vi "Autonomous Independent.vi"   [LabVIEW 2015]
doc: "This VI is called when autonomous begins, and will automatically be terminated when autonomous ends. You can carry out timed or sensor driven robot movement independently without needing to return to the caller."
uses:
  <vilib>/Rock Robotics/WPI/Solenoid/WPI_SolenoidValue.ctl
  <vilib>/Rock Robotics/WPI/Utilities/WPI_GetSetVariantRefNum.vi
  <vilib>/Rock Robotics/Network Tables/NT Read String.vi
  <vilib>/Rock Robotics/Network Tables/NT Read Number.vi
  <vilib>/Rock Robotics/WPI/Solenoid/WPI_SolenoidSetEnum.vi
  <vilib>/Rock Robotics/Network Tables/NT Write Numeric Array.vi
panel:
  # "Be sure to right-click and choose Data Operations>>Make Current Value default if you want to save the array values with the VI"
types:
  T1 = typedef "WPI_JoystickDevRef.ctl" = cluster{"Device":T2}
  T2 = typedef "WPI_JoystickDeviceEnum.ctl" = enum16{"USB 0", "USB 1", "USB 2", "USB 3", "USB 4", "USB 5"}
  T3 = typedef "WPI_ServoDeviceRef.ctl" = cluster{"DeviceStatus":errorcluster, "PWM Channel":T4, "DeadBand":T5}
  T4 = typedef "FPGA_DIOPWMChannel.ctl" = enum8{"PWM 0", "PWM 1", "PWM 2", "PWM 3", "PWM 4", "PWM 5", "PWM 6", "PWM 7", "PWM 8", "PWM 9", "PWM MXP 0", "PWM MXP 1", "PWM MXP 2", "PWM MXP 3", "PWM MXP 4", "PWM MXP 5", "PWM MXP 6", "PWM MXP 7", "PWM MXP 8", "PWM MXP 9", "Invalid"}
  T5 = typedef "WPI_PWMDeadband.ctl" = cluster{"Name":string, "maxPositivePwm":i32, "minPositivePwm":i32, "centerPwm":i32, "maxNegativePwm":i32, "minNegativePwm":i32, "angularRange":u16}
  T6 = typedef "WPI_SolenoidValue.ctl" = enum16{"Off", "On", "Forward", "Reverse"}
  T7 = typedef "WPI_SwitchDevRef.ctl" = cluster{"DevStatus":errorcluster, "DIO Channel":T8, "CntIndex":T9, "Normally Closed":bool}
  T8 = typedef "FPGA_DIOChannel.ctl" = enum8{"DIO 0", "DIO 1", "DIO 2", "DIO 3", "DIO 4", "DIO 5", "DIO 6", "DIO 7", "DIO 8", "DIO 9", "DIO MXP 0", "DIO MXP 1", "DIO MXP 2", "DIO MXP 3", "DIO MXP 4", "DIO MXP 5", "DIO MXP 6", "DIO MXP 7", "DIO MXP 8", "DIO MXP 9", "DIO MXP 10", "DIO MXP 11", "DIO MXP 12", "DIO MXP 13", "DIO MXP 14", "DIO MXP 15", "Invalid"}
  T9 = typedef "FPGA_CounterCtrSystemIndex.ctl" = enum8{"Ctr 0", "Ctr 1", "Ctr 2", "Ctr 3", "Ctr 4", "Ctr 5", "Ctr 6", "Ctr 7", "Invalid"}
  T10 = typedef "WPI_SolenoidDevRef.ctl" = cluster{"DevStatus":errorcluster, "Pneumatics Control Module":u8, "Forward Solenoid Channel":T11, "Reverse Solenoid Channel":T11}
  T11 = typedef "WPI_SolenoidChannel.ctl" = enum8{"Solenoid 0", "Solenoid 1", "Solenoid 2", "Solenoid 3", "Solenoid 4", "Solenoid 5", "Solenoid 6", "Solenoid 7", "Invalid"}
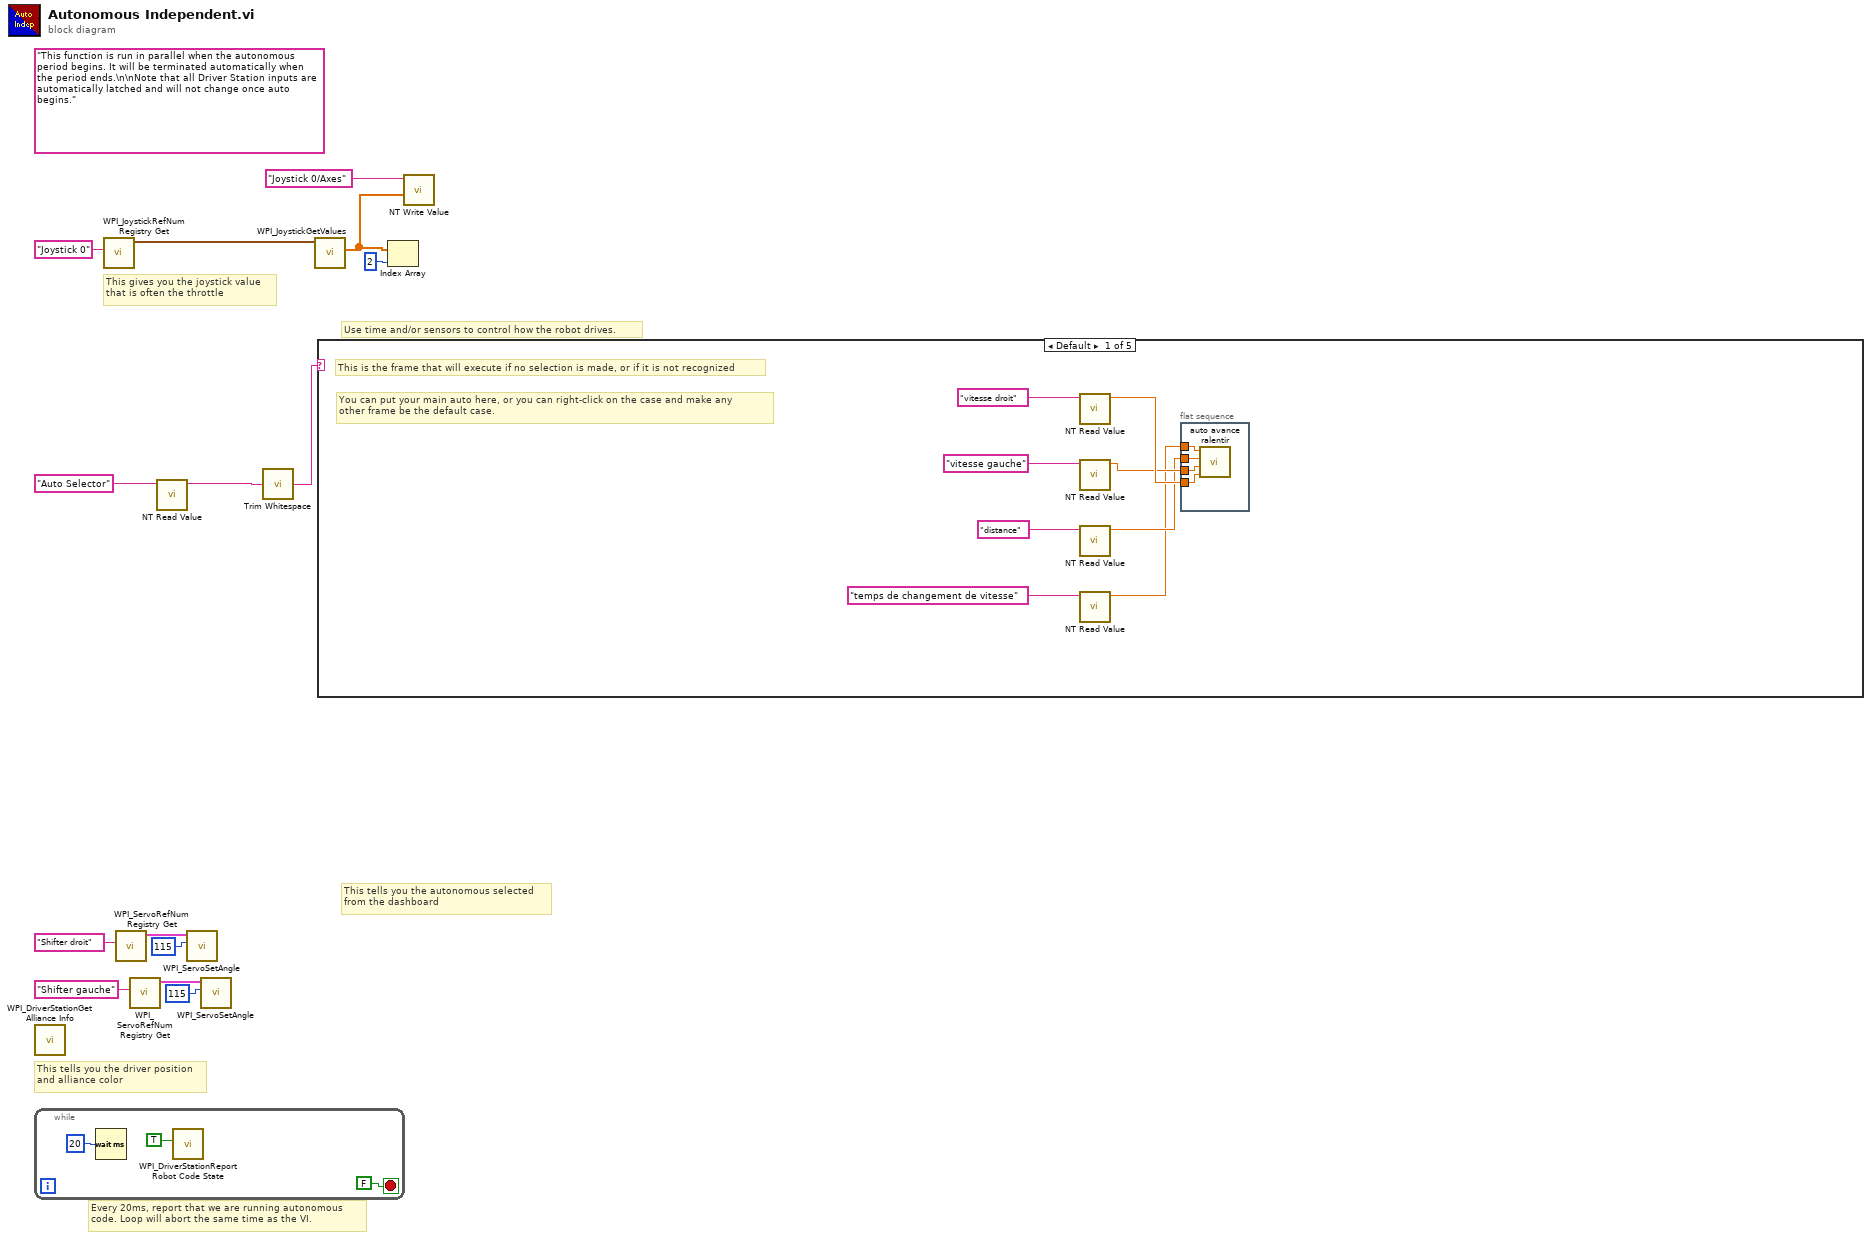
[diagram p0: block diagram]
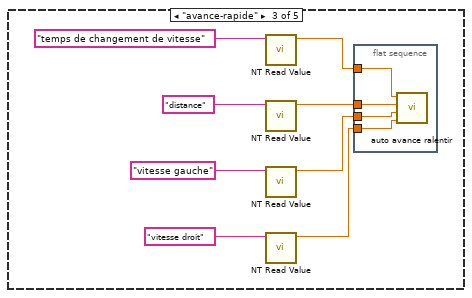
[diagram p3: hidden frame]
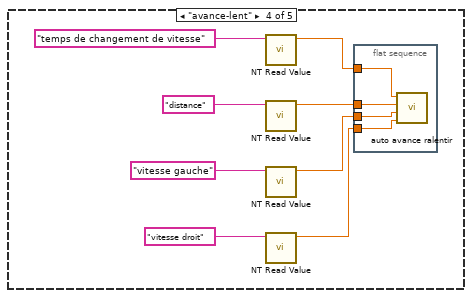
[diagram p4: hidden frame]
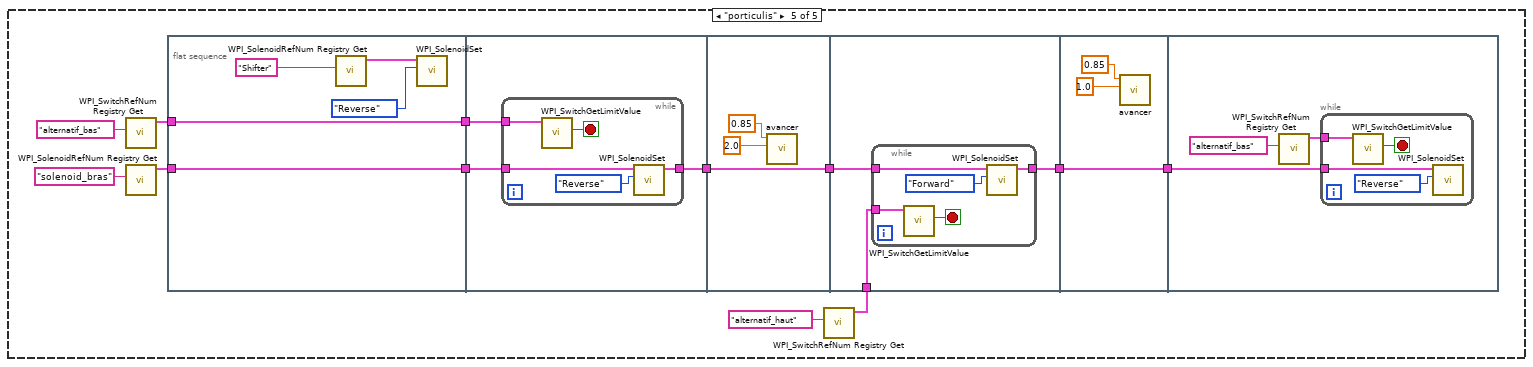
[diagram p5: hidden frame]
diagram:
  (unwired) "This function is run in parallel when the autonomous period begins. It will be terminated automatically when the period ends.\n\nNote that all Driver Station inputs are automatically latched and will not change once auto begins."
  # "This tells you the autonomous selected\nfrom the dashboard"
  # "Every 20ms, report that we are running autonomous\ncode. Loop will abort the same time as the VI."
  # "This gives you the joystick value\nthat is often the throttle"
  # "Use time and/or sensors to control how the robot drives."
  # "This tells you the driver position\nand alliance color"
  n1 = call <vilib>:"WPI_DriverStationGet Alliance Info.vi"() -> ()  [unwired: 12 out]
  n2 = while {
    stop <- FALSE stop-if-true
    n3 = Wait (ms)(milliseconds to wait=u32 20) -> ()  [unwired: 1 out]
    n4 = call <vilib>:"WPI_DriverStationReport Robot Code State.vi"("Autonomous"=TRUE) -> ()  [unwired: 10 in, 1 out]
  }
  n5 = call <vilib>:"WPI_JoystickRefNum Registry Get.vi"("refnum name"="Joystick 0") -> ("JoystickDevRef"=w13:T1)  [unwired: 1 in, 9 out]
  n6 = call <vilib>:"WPI_ServoRefNum Registry Get.vi"("refnum name"="Shifter droit") -> ("ServoDeviceRef"=w5:T3)  [unwired: 9 in, 1 out]
  n7 = call <vilib>:"WPI_ServoRefNum Registry Get.vi"("refnum name"="Shifter gauche") -> ("ServoDeviceRef"=w3:T3)  [unwired: 9 in, 1 out]
  n8 = call-poly <vilib>:"NT Read Value.vi"("Name"="Auto Selector") -> ("String"=w1:string)  [unwired: 9 in, 1 out]
  n9 = call <vilib>:"WPI_ServoSetAngle.vi"("Angle"=115, "ServoDeviceRef"=w5) -> ()  [unwired: 8 in, 2 out]
  n10 = call <vilib>:"WPI_ServoSetAngle.vi"("Angle"=115, "ServoDeviceRef"=w3) -> ()  [unwired: 8 in, 2 out]
  n11 = call <vilib>:"Trim Whitespace.vi"("string"=w1) -> ("trimmed string"=w2:string)  [unwired: 1 in]
  n12 = call <vilib>:"WPI_JoystickGetValues.vi"("JoystickDevRef"=w13) -> ("Axes"=w10:dbl[])  [unwired: 6 in, 4 out]
  n13 = case shown="Default" w2 {
    frame Default {
      # "You can put your main auto here, or you can right-click on the case and make any\nother frame be the default case."
      # "This is the frame that will execute if no selection is made, or if it is not recognized"
      n14 = call-poly <vilib>:"NT Read Value.vi"("Name"="vitesse droit") -> ("Numeric"=w21:dbl)  [unwired: 9 in, 1 out]
      n15 = call-poly <vilib>:"NT Read Value.vi"("Name"="vitesse gauche") -> ("Numeric"=w20:dbl)  [unwired: 9 in, 1 out]
      n16 = call-poly <vilib>:"NT Read Value.vi"("Name"="distance") -> ("Numeric"=w19:dbl)  [unwired: 9 in, 1 out]
      n17 = call-poly <vilib>:"NT Read Value.vi"("Name"="temps de changement de vitesse") -> ("Numeric"=w18:dbl)  [unwired: 9 in, 1 out]
      n18 = flat-sequence {
        tunnel: w18 -> [w29]
        tunnel: w20 -> [w27]
        tunnel: w21 -> [w26]
        tunnel: w19 -> [w28]
        frame #0 {
          n19 = call "auto avance ralentir.vi"("vitesse droit"=w26, "vitesse gauche"=w27, "temps"=w28, "temps de changement de direction"=w29) -> ()  [unwired: 8 in]
        }
      }
    }
    frame "rien" {
    }
    frame "avance-rapide" {
      n20 = call-poly <vilib>:"NT Read Value.vi"("Name"="temps de changement de vitesse") -> ("Numeric"=w30:dbl)  [unwired: 9 in, 1 out]
      n21 = call-poly <vilib>:"NT Read Value.vi"("Name"="distance") -> ("Numeric"=w31:dbl)  [unwired: 9 in, 1 out]
      n22 = call-poly <vilib>:"NT Read Value.vi"("Name"="vitesse gauche") -> ("Numeric"=w32:dbl)  [unwired: 9 in, 1 out]
      n23 = call-poly <vilib>:"NT Read Value.vi"("Name"="vitesse droit") -> ("Numeric"=w33:dbl)  [unwired: 9 in, 1 out]
      n24 = flat-sequence {
        tunnel: w30 -> [w41]
        tunnel: w32 -> [w39]
        tunnel: w33 -> [w38]
        tunnel: w31 -> [w40]
        frame #0 {
          n25 = call "auto avance ralentir.vi"("vitesse droit"=w38, "vitesse gauche"=w39, "temps"=w40, "temps de changement de direction"=w41) -> ()  [unwired: 8 in]
        }
      }
    }
    frame "avance-lent" {
      n26 = call-poly <vilib>:"NT Read Value.vi"("Name"="temps de changement de vitesse") -> ("Numeric"=w42:dbl)  [unwired: 9 in, 1 out]
      n27 = call-poly <vilib>:"NT Read Value.vi"("Name"="distance") -> ("Numeric"=w43:dbl)  [unwired: 9 in, 1 out]
      n28 = call-poly <vilib>:"NT Read Value.vi"("Name"="vitesse gauche") -> ("Numeric"=w44:dbl)  [unwired: 9 in, 1 out]
      n29 = call-poly <vilib>:"NT Read Value.vi"("Name"="vitesse droit") -> ("Numeric"=w45:dbl)  [unwired: 9 in, 1 out]
      n30 = flat-sequence {
        tunnel: w42 -> [w53]
        tunnel: w44 -> [w51]
        tunnel: w45 -> [w50]
        tunnel: w43 -> [w52]
        frame #0 {
          n31 = call "auto avance ralentir.vi"("vitesse droit"=w50, "vitesse gauche"=w51, "temps"=w52, "temps de changement de direction"=w53) -> ()  [unwired: 8 in]
        }
      }
    }
    frame "porticulis" {
      n32 = call <vilib>:"WPI_SwitchRefNum Registry Get.vi"("refnum name"="alternatif_bas") -> ("SwitchDevRef"=w65:T7)  [unwired: 9 in, 1 out]
      n33 = call <vilib>:"WPI_SolenoidRefNum Registry Get.vi"("refnum name"="solenoid_bras") -> ("SolenoidDevRef"=w62:T10)  [unwired: 9 in, 1 out]
      n34 = flat-sequence {
        tunnel: w62 -> [w69]
        tunnel: w65 -> [w70]
        tunnel: [w70] -> w56
        tunnel: [w69] -> w55
        tunnel: [w71] -> w59
        tunnel: w56 -> [w73]
        tunnel: w55 -> [w72]
        tunnel: [w81] -> w60
        tunnel: w59 -> [w81]
        tunnel: w63 -> [w84]
        tunnel: w60 -> [w83]
        tunnel: [w82] -> w58
        tunnel: w58 -> [w92]
        tunnel: [w92] -> w57
        tunnel: w57 -> [w95]
        frame #0 {
          n35 = call <vilib>:"WPI_SolenoidRefNum Registry Get.vi"("refnum name"="Shifter") -> ("SolenoidDevRef"=w68:T10)  [unwired: 9 in, 1 out]
          n36 = call-poly <vilib>:"WPI_SolenoidSet.vi"("Value"=WPI_SolenoidValue."Reverse", "SolenoidDevRef"=w68) -> ()  [unwired: 8 in, 2 out]
        }
        frame #1 {
          n37 = while {
            tunnel: w73 -> [w78]
            tunnel: w72 -> [w76]
            tunnel: [w74] -> w71
            stop <- w77 stop-if-true
            n38 = call <vilib>:"WPI_SwitchGetLimitValue.vi"("SwitchDevRef"=w78) -> ("Switch Pressed"=w77:bool)  [unwired: 8 in, 2 out]
            n39 = call-poly <vilib>:"WPI_SolenoidSet.vi"("Value"=WPI_SolenoidValue."Reverse", "SolenoidDevRef"=w76) -> ("SolenoidDevRef"=w74:T10)  [unwired: 8 in, 1 out]
          }
        }
        frame #2 {
          n40 = call "avancer.vi"("Distance"=2.0, "Vitesse"=0.85) -> ()  [unwired: 10 in]
        }
        frame #3 {
          n41 = while {
            tunnel: w84 -> [w89]
            tunnel: w83 -> [w87]
            tunnel: [w85] -> w82
            stop <- w88 stop-if-true
            n42 = call <vilib>:"WPI_SwitchGetLimitValue.vi"("SwitchDevRef"=w89) -> ("Switch Pressed"=w88:bool)  [unwired: 8 in, 2 out]
            n43 = call-poly <vilib>:"WPI_SolenoidSet.vi"("Value"=WPI_SolenoidValue."Forward", "SolenoidDevRef"=w87) -> ("SolenoidDevRef"=w85:T10)  [unwired: 8 in, 1 out]
          }
        }
        frame #4 {
          n44 = call "avancer.vi"("Distance"=1.0, "Vitesse"=0.85) -> ()  [unwired: 10 in]
        }
        frame #5 {
          n45 = call <vilib>:"WPI_SwitchRefNum Registry Get.vi"("refnum name"="alternatif_bas") -> ("SwitchDevRef"=w94:T7)  [unwired: 9 in, 1 out]
          n46 = while {
            tunnel: w95 -> [w99]
            tunnel: w94 -> [w96]
            stop <- w97 stop-if-true
            n47 = call <vilib>:"WPI_SwitchGetLimitValue.vi"("SwitchDevRef"=w96) -> ("Switch Pressed"=w97:bool)  [unwired: 8 in, 2 out]
            n48 = call-poly <vilib>:"WPI_SolenoidSet.vi"("Value"=WPI_SolenoidValue."Reverse", "SolenoidDevRef"=w99) -> ()  [unwired: 8 in, 2 out]
          }
        }
      }
      n49 = call <vilib>:"WPI_SwitchRefNum Registry Get.vi"("refnum name"="alternatif_haut") -> ("SwitchDevRef"=w63:T7)  [unwired: 9 in, 1 out]
    }
  }
  n50 = Index Array(array=w10, index=2) -> ()  [unwired: 1 out]
  n51 = call-poly <vilib>:"NT Write Value.vi"("Numeric Array"=w10, "Name"="Joystick 0/Axes") -> ()  [unwired: 9 in, 1 out]
